vi "Retriggerable Analog Input (STC2).vi"() -> ()   [LabVIEW 2009]
doc: "I. Description:\nThis example demonstrates how to generate a finite digital pulse train from a Counter Output Channel. And use the pulse train as the clock source for an analog input operation."
uses:
  <vilib>/DAQmx/create/channels.llb/DAQmx Create Channel (CO-Pulse Generation-Frequency).vi
  <vilib>/DAQmx/configure/timing.llb/DAQmx Timing (Implicit).vi
  Program Files/National Instruments/LabVIEW 2009/resource/objmgr/daqmx.rc
  <vilib>/DAQmx/configure/trigger.llb/DAQmx Start Trigger (Digital Edge).vi
  <vilib>/DAQmx/create/channels.llb/DAQmx Create Channel (AI-Voltage-Basic).vi
panel:
  in  "analog input channels":tag="Dev1/ai2"
  in  "samples per channel":i32=10
  in  "stop":bool
  out "data":dbl[](graph)=[0.11633395532614343, 2.322477792337649, 2.49304052741351, 2.4512898694732237, 0.7765741109067276, -1.6028776767751645, -2.866070770695397, -2.8212456872470555, -1.0924868869830124, 1.3269366026043294]
  in  "initial delay":dbl format="%.6f"
  in  "idle state":i32(ring)=10214 items=["High"=10192, "Low"=10214]
  in  "counter":tag="Dev1/ctr0"
  in  "frequency":dbl=10.0 format="%.6f"
  in  "duty cycle":dbl=0.5 format="%.6f"
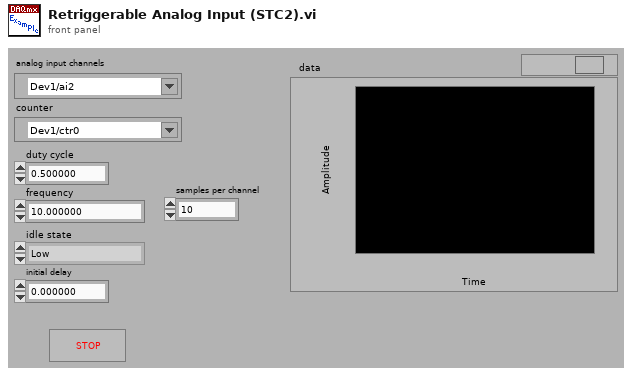
[diagram p1: front panel]
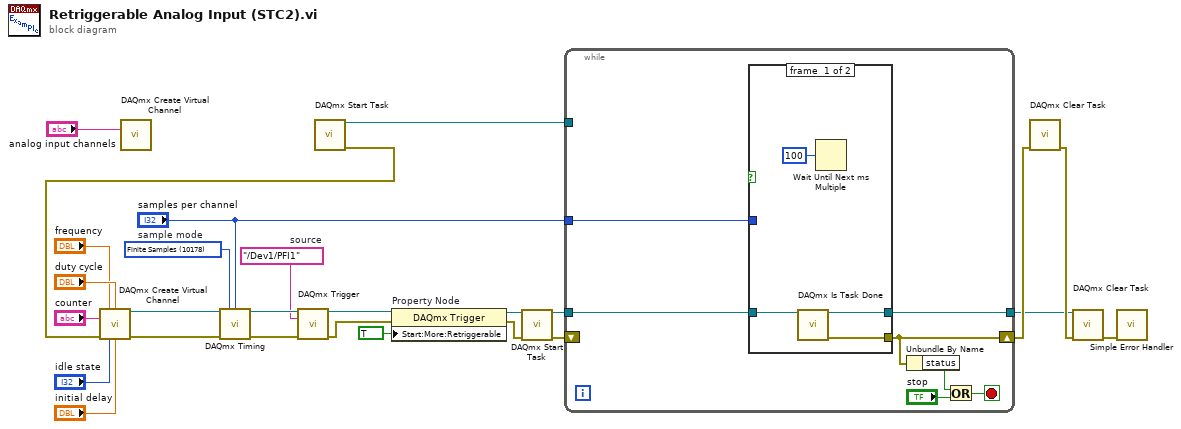
[diagram p0: block diagram]
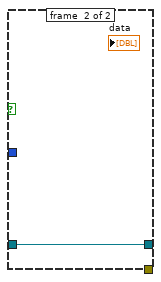
[diagram p2: hidden frame]
diagram:
  w14 = tag "/Dev1/PFI1"  # source
  w17 = 10178 items=["Finite Samples"=10178, "Continuous Samples"=10123]  # sample mode
  n1 = call-poly <vilib>:"DAQmx Create Virtual Channel.vi"("physical channels"="analog input channels") -> ()  [unwired: 13 in, 2 out]
  n2 = call <vilib>:"DAQmx Start Task.vi"() -> ("task out"=w8:refnum<k21>, "error out"=w7:errorcluster)  [unwired: 14 in]
  n3 = call-poly <vilib>:"DAQmx Create Virtual Channel.vi"("frequency"="frequency", "duty cycle"="duty cycle", "counter"="counter", "error in"=w7, "idle state"="idle state", "initial delay"="initial delay") -> ("task out"=w19:refnum<k21>, "error out"=w18:errorcluster)  [unwired: 8 in]
  n4 = call-poly <vilib>:"DAQmx Timing.vi"("task/channels in"=w19, "sample mode"=w17, "samples per channel"="samples per channel", "error in"=w18) -> ("task out"=w16:refnum<k21>, "error out"=w15:errorcluster)  [unwired: 10 in]
  n5 = call-poly <vilib>:"DAQmx Trigger.vi"("task/channels in"=w16, "source"=w14, "error in"=w15) -> ("task out"=w13:refnum<k21>, "error out"=w12:errorcluster)  [unwired: 11 in]
  n6 = property on="Property Node" class="DAQmx Trigger"(reference=w13, error in=w12, "Start:More:Retriggerable"=TRUE ("Start.Retriggerable")) -> (reference out=w10:refnum<k21>, error out=w9:errorcluster)
  n7 = call <vilib>:"DAQmx Start Task.vi"("task/channels in"=w10, "error in"=w9) -> ("task out"=w22:refnum<k21>, "error out"=w21:errorcluster)  [unwired: 12 in]
  n8 = while {
    tunnel: w22 -> [w30]
    tunnel: [w29] -> w3
    shift-right: [w28] -> w5
    shift-left: w21 -> [_]
    tunnel: w8 -> [_]
    tunnel: "samples per channel" -> [w27]
    stop <- w31 stop-if-true
    n9 = case shown="False" {
      selector: _ -> [_ _]
      tunnel: w30 -> [w36 w38]
      tunnel: [w35 w38] -> w29
      tunnel: [w34 _] -> w28
      tunnel: w27 -> [_ _]
      frame #0 {
        n10 = call <vilib>:"DAQmx Is Task Done.vi"("task/channels in"=w36) -> ("task out"=w35:refnum<k21>, "error out"=w34:errorcluster)  [unwired: 12 in, 1 out]
        n11 = Wait Until Next ms Multiple(millisecond multiple=u32 100) -> ()  [unwired: 1 out]
      }
      frame #1 {
      }
    }
    n12 = Unbundle By Name "Unbundle By Name"(w28) -> ("status"=w33:bool)
    n13 = Or(x=w33, y="stop") -> (x .or. y?=w31:bool)
  }
  n14 = call <vilib>:"DAQmx Clear Task.vi"("error in"=w5) -> ("error out"=w4:errorcluster)  [unwired: 14 in]
  n15 = call <vilib>:"DAQmx Clear Task.vi"("task in"=w3, "error in"=w4) -> ("error out"=w20:errorcluster)  [unwired: 13 in]
  n16 = call <vilib>:"Simple Error Handler.vi"("error in (no error)"=w20) -> ()  [unwired: 4 in, 5 out]
